vi "MX1 Contactor Test.vi"(8 "error in (no error)":errorcluster, 10 "Message IN":string) -> (0 "error out":errorcluster, 1 "Result (bool)":bool, 2 "Message OUT":string, 3 "VISA resource name 2":refnum<visa-resource-name>)   [LabVIEW 2022 SP3]
panel:
  in  "BYPASS":bool
  in  "FAIL":bool
  in  "PASS":bool
  in  "Main AC Contactor":bool
  out "Result (color)":u32(colorbox)
  # "Toggle the main AC contactor. Does it open and close as expected?"
  # "Off = Open\nOn = Closed"
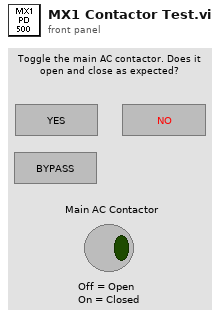
[diagram p1: front panel]
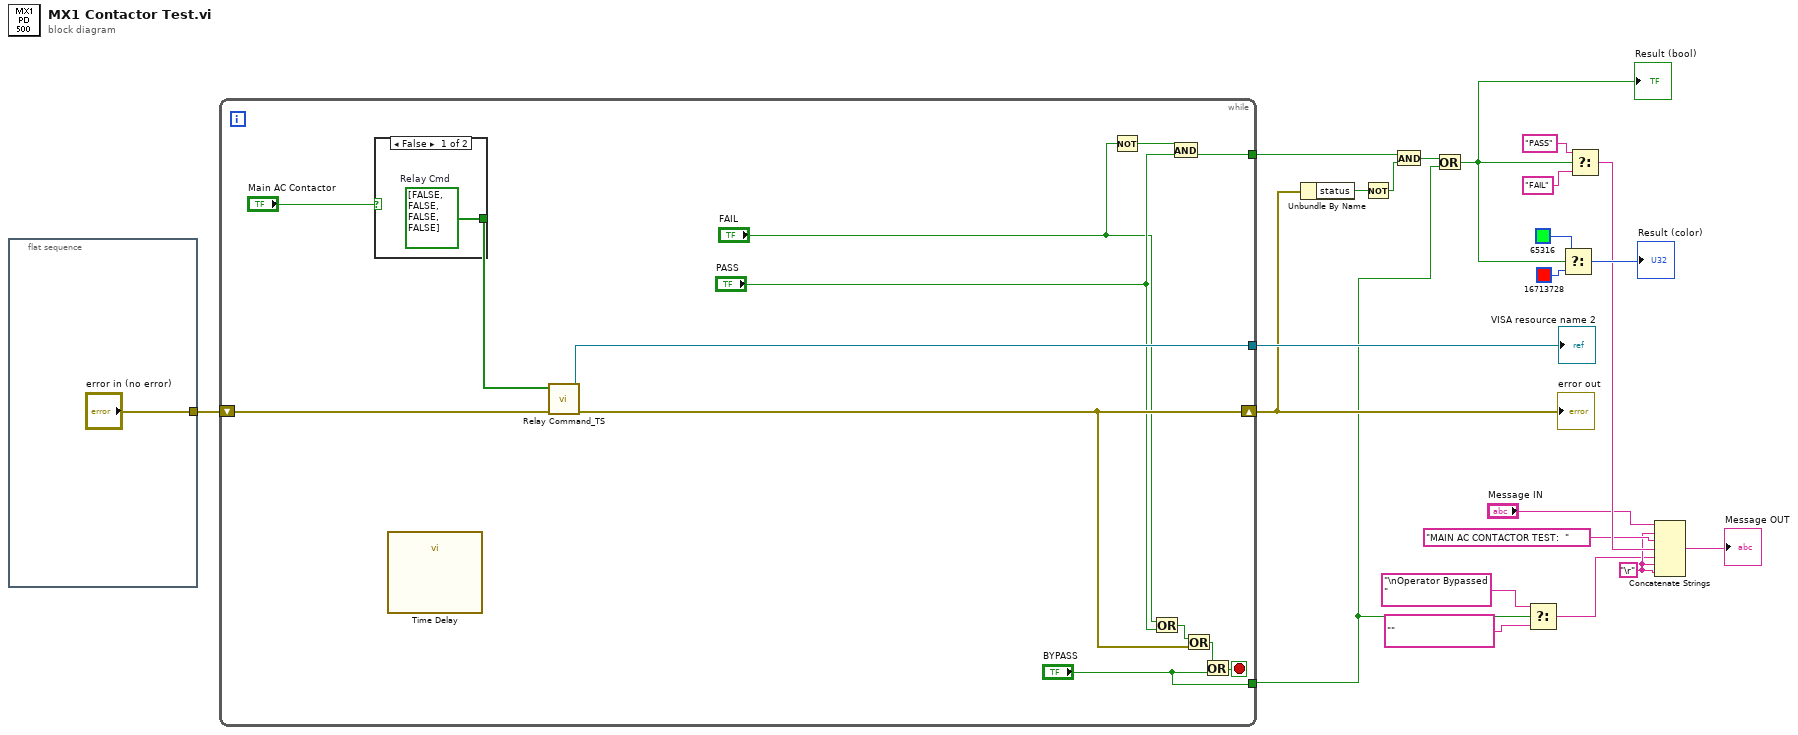
[diagram p0: block diagram]
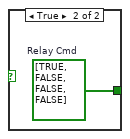
[diagram p2: hidden frame]
diagram:
  w9 = "\r"
  n1 = flat-sequence {
    tunnel: ["error in (no error)"] -> w19
    frame #0 {
    }
  }
  n2 = while {
    shift-right: [w33] -> w7
    shift-left: w19 -> [w36]
    tunnel: [w35] -> w22
    tunnel: [w29] -> w8
    tunnel: ["BYPASS"] -> w3
    stop <- w26 stop-if-true
    n3 = case shown="False" "Main AC Contactor" {
      tunnel: [w37 w38] -> w24
      frame False {
        w37 = bool[] [FALSE, FALSE, FALSE, FALSE]  # Relay Cmd
      }
      frame True {
        w38 = bool[] [TRUE, FALSE, FALSE, FALSE]  # Relay Cmd
      }
    }
    n4 = call "Time Delay"() -> ()  [unwired: 11 in, 1 out]
    n5 = call "Relay Command_TS.vi"("error in (no error)"=w36, "Relay Command"=w24) -> ("error out"=w33:errorcluster, "VISA Refnum out"=w35:refnum<visa-resource-name>)  [unwired: 8 in]
    n6 = Not(x="FAIL") -> (.not. x?=w28:bool)
    n7 = Or(x="FAIL", y="PASS") -> (x .or. y?=w32:bool)
    n8 = And(x=w28, y="PASS") -> (x .and. y?=w29:bool)
    n9 = Or(x=w32, y=w33) -> (x .or. y?=w31:bool)
    n10 = Or(x=w31, y="BYPASS") -> (x .or. y?=w26:bool)
  }
  "error out" <- w7
  "VISA resource name 2" <- w22
  n11 = Unbundle By Name(w7) -> ("status"=w15:bool)
  n12 = Not(x=w15) -> (.not. x?=w14:bool)
  n13 = And(x=w8, y=w14) -> (x .and. y?=w5:bool)
  n14 = Or(x=w5, y=w3) -> (x .or. y?=w6:bool)
  "Result (bool)" <- w6
  n15 = Select(t="\nOperator Bypassed ", s=w3, f="") -> (s? t:f=w4:string)
  n16 = Select(t=u32 65316 ("Result (color)"), s=w6, f=u32 16713728 ("Result (color)")) -> (s? t:f=→"Result (color)":u32)
  n17 = Select(t="PASS", s=w6, f="FAIL") -> (s? t:f=w12:string)
  n18 = Concatenate Strings("Message IN", w9, "MAIN AC CONTACTOR TEST:  ", w12, w4, w9, w9) -> (→"Message OUT":string)
